vi "Image_Detect_Object.vi"(0 "Data":T3={"system"={"info"={"menuSelect"=0, "version"=0, "serial"="Test Sample", "captureActive"=FALSE, "captureBegin"=FALSE, "emptyAndRefill"=FALSE}, "userInfo"={"operatorName"="MRJ", "date"=timestamp(2713993200 s since 1904-01-01)}, "camera"={"exposureTime"=1, "aperture"=enum."Item 0", "framerate"=1, "framerateMax"=500, "legacyAttributes"=FALSE}}, "connections"={"arduino"={"connection"="MRJ", "status"=FALSE, "openState"=FALSE, "emptyStart"=500}, "pump"={"connection"="MRJ", "status"=FALSE, "command"="", "dispenseSpeed"=500, "flushSize"=100}, "camera"={"cam1"={"connection"="", "status"=FALSE}, "cam2"={"connection"="", "status"=FALSE}}}, "queue"={"process"={"cam1"=refnum, "cam2"=refnum, "queueSize"=0}, "save"={"cam1"=refnum, "cam2"=refnum, "queueSize"=0}, "overloadThreshold"=0}, "imageProcess"={"cam1"={"preAllocation"={"image"="Station", "originalDisplay"="Station", "originalRgb"="Station", "binary"="Station", "save"="Station", "calibrationFull"=refnum, "calibrationDetect"=refnum}, "calibration"={"pathFull"=path "C:/Users/au540322/Desktop/IHS_Project/images/Debris/Debris_0/Debris_0_2019_06_01-23-32-49-686.PNG", "pathDetect"=path "C:/Users/au540322/Desktop/IHS_Project/images/Debris/Debris_0/Debris_0_2019_06_01-23-32-49-686.PNG", "ROI"={"Left"=0, "Top"=0, "Right"=0, "Bottom"=0, "Rotation"=0.0}}}, "cam2"={"preAllocation"={"image"=refnum, "originalDisplay"=refnum, "originalRgb"=refnum, "binary"=refnum, "save"=refnum, "calibrationFull"=refnum, "calibrationDetect"=refnum}, "calibration"={"pathFull"=path "C:/Users/au540322/Desktop/IHS_Project/images/Debris/Debris_0/Debris_0_2019_06_01-23-32-49-686.PNG", "pathDetect"=path "C:/Users/au540322/Desktop/IHS_Project/images/Debris/Debris_0/Debris_0_2019_06_01-23-32-49-686.PNG", "ROI"={"Left"=0, "Top"=100, "Right"=100, "Bottom"=0, "Rotation"=0.0}}}, "process"={"planeExtract"=refnum, "planeSubtract"=refnum, "cropMask"=refnum}, "detection"={"sampleTimeout"=200, "sizeThreshold"=500, "detectionRegionPct"=0.0}}, "sampleData"={"sampleId"="", "projectId"="", "voucherID"="", "speciesName"="", "collectionDate"=timestamp(2713993200 s since 1904-01-01), "sampleStation"="", "location"="", "lat"=0.0, "lon"=0.0, "determiner"="", "sex"="", "otherNotes"=""}, "Session In"=""} {"sampleData"."collectionDate" format="%<%Y-%m-%d>T"; "imageProcess"."detection"."sizeThreshold" min=1; "imageProcess"."cam2"."calibration"."ROI"."Rotation" format="%.2f"; "imageProcess"."cam2"."calibration"."ROI"."Left" scale=0.0..1024.0; "imageProcess"."cam2"."calibration"."ROI"."Right" scale=0.0..1024.0; "imageProcess"."cam1"."calibration"."ROI"."Rotation" format="%.2f"; "imageProcess"."cam1"."calibration"."ROI"."Left" scale=0.0..1024.0; "imageProcess"."cam1"."calibration"."ROI"."Right" scale=0.0..1024.0; "queue"."overloadThreshold" min=1; "queue"."save"."queueSize" min=1; "queue"."process"."queueSize" min=1; "connections"."pump"."flushSize" min=1; "connections"."pump"."dispenseSpeed" min=1; "system"."camera"."framerateMax" min=1; "system"."userInfo"."date" format="%<%Y-%m-%dT%H:%M:%S+%z>T"; "system"."info"."version" items=["Standard", "XL"]; "system"."info"."menuSelect" items=["Session Data", "Extended Setup", "Buffer", "Camera", "Dispenser", "Stats", "Connections"]}, 5 "Image Pixels (U32)":u32[][](array[numeric]), 9 "Detect Crop":bool, 12 "Camera":T6=enum."Camera 2") -> (2 "error out":errorcluster, 3 "Obj Size":bool, 4 "Crop Image Out":T1(plugin-control), 6 "New image":T1(plugin-control), 8 "Image Binary":T1(plugin-control), 10 "Object Accept":bool, 14 "ROI descriptor":T2, 15 "Sample Data":dbl[](array[numeric]))   [LabVIEW 2022 SP3]
uses:
  <vilib>/vision/NI_Vision_Development_Module.lvlib
  Camera_ID.ctl
  <vilib>/userdefined/High Color/IMAQdx.ctl
  <vilib>/vision/Image Controls.llb/IMAQ Image.ctl
  controls/Data.ctl
panel:
  out "New image Blue plane":T1(plugin-control)
  out "Subtract":T1(plugin-control)
  in  "error in":errorcluster
  in  "Threshold":cluster{"Lower value":sgl, "Upper value":sgl}={"Lower value"=15.0, "Upper value"=256.0} {"Upper value" format="%.2f"; "Lower value" format="%.2f"}
  out "Calibration image in":T1(plugin-control)
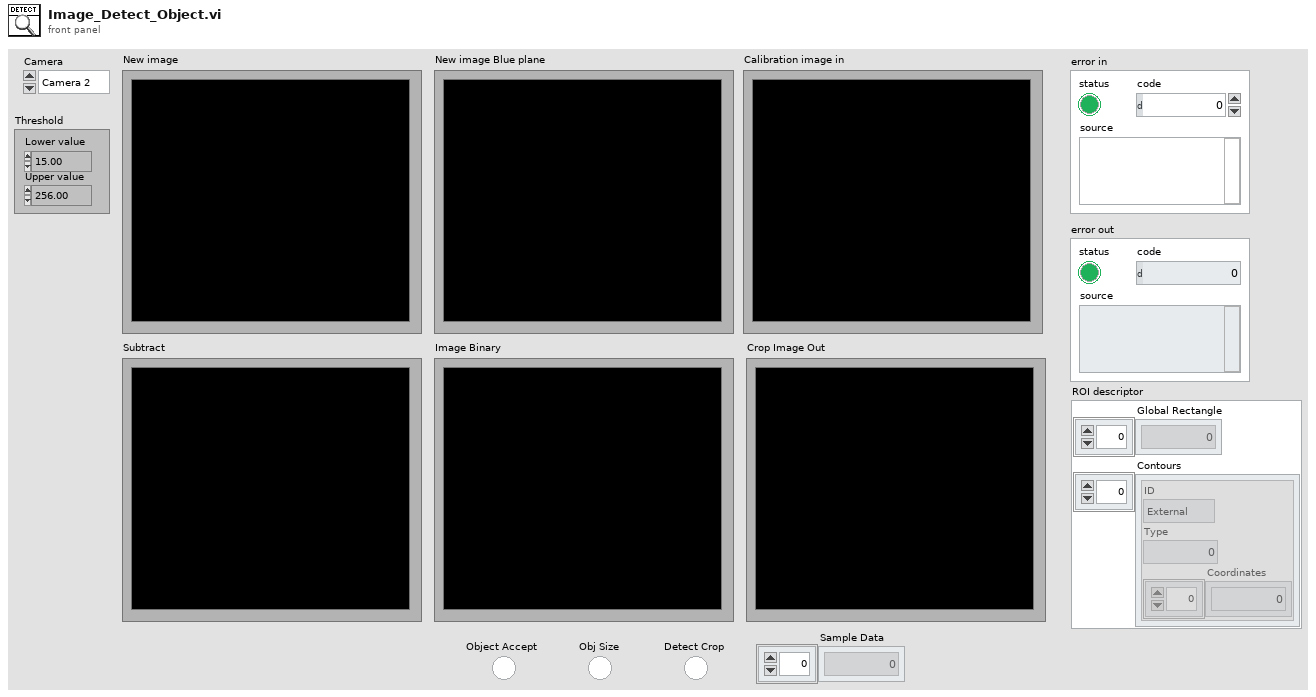
[diagram p1: front panel]
types:
  T1 = typedef "IMAQ Image.ctl" = refnum<image>
  T2 = cluster{"Global Rectangle":i32[], "Contours":cluster{"ID":enum32{"External", "Internal"}, "Type":u32, "Coordinates":i32[]}[]}
  T3 = typedef "Data.ctl" = cluster{"system":cluster{"info":cluster{"menuSelect":u16, "version":u16, "serial":string, "captureActive":bool, "captureBegin":bool, "emptyAndRefill":bool}, "userInfo":cluster{"operatorName":string, "date":timestamp}, "camera":cluster{"exposureTime":i32, "aperture":enum32{"Item 0", "Item 1", "Item 2", "Item 3"}, "framerate":i32, "framerateMax":i32, "legacyAttributes":bool}}, "connections":cluster{"arduino":cluster{"connection":refnum<visa-resource-name>, "status":bool, "openState":bool, "emptyStart":u32}, "pump":cluster{"connection":refnum<visa-resource-name>, "status":bool, "command":string, "dispenseSpeed":i32, "flushSize":i32}, "camera":cluster{"cam1":cluster{"connection":T4, "status":bool}, "cam2":cluster{"connection":T4, "status":bool}}}, "queue":cluster{"process":cluster{"cam1":refnum<queue>, "cam2":refnum<queue>, "queueSize":i32}, "save":cluster{"cam1":refnum<queue>, "cam2":refnum<queue>, "queueSize":i32}, "overloadThreshold":i32}, "imageProcess":cluster{"cam1":cluster{"preAllocation":cluster{"image":T1, "originalDisplay":T1, "originalRgb":T1, "binary":T1, "save":T1, "calibrationFull":T1, "calibrationDetect":T1}, "calibration":cluster{"pathFull":path, "pathDetect":path, "ROI":T5}}, "cam2":cluster{"preAllocation":cluster{"image":T1, "originalDisplay":T1, "originalRgb":T1, "binary":T1, "save":T1, "calibrationFull":T1, "calibrationDetect":T1}, "calibration":cluster{"pathFull":path, "pathDetect":path, "ROI":T5}}, "process":cluster{"planeExtract":T1, "planeSubtract":T1, "cropMask":T1}, "detection":cluster{"sampleTimeout":i32, "sizeThreshold":i32, "detectionRegionPct":dbl}}, "sampleData":cluster{"sampleId":string, "projectId":string, "voucherID":string, "speciesName":string, "collectionDate":timestamp, "sampleStation":string, "location":string, "lat":dbl, "lon":dbl, "determiner":string, "sex":string, "otherNotes":string}, "Session In":T4}
  T4 = typedef "IMAQdx.ctl" = refnum<k21>
  T5 = typedef "IMAQ Rectangle" = cluster{"Left":i32, "Top":i32, "Right":i32, "Bottom":i32, "Rotation":dbl}
  T6 = typedef "Camera_ID.ctl" = enum16{"Camera 1", "Camera 2"}
  T7 = typedef "Particle Parameters" = i32
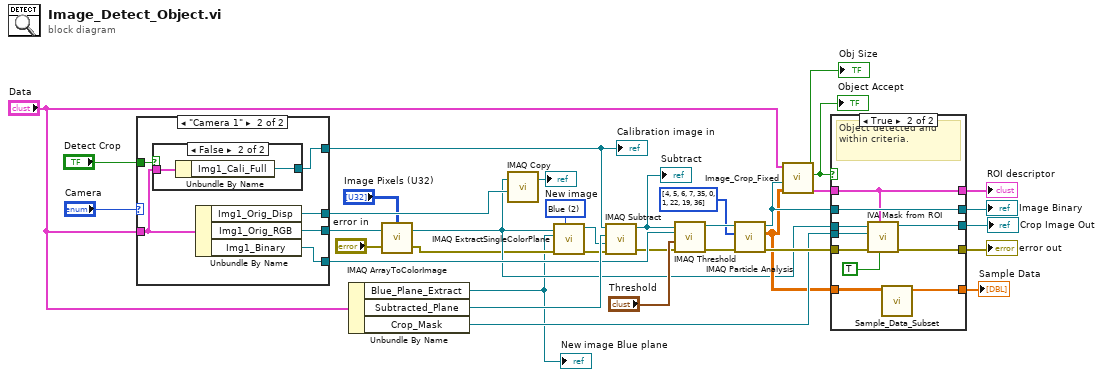
[diagram p0: block diagram]
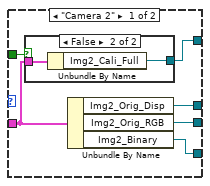
[diagram p2: hidden frame]
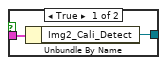
[diagram p3: hidden frame]
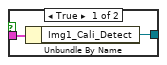
[diagram p4: hidden frame]
diagram:
  w17 = T7[] [4, 5, 6, 7, 35, 0, 1, 22, 19, 36] items=["Center of Mass X", "Center of Mass Y", "First Pixel X", "First Pixel Y", "Bounding Rect Left", "Bounding Rect Top", "Bounding Rect Right", "Bounding Rect Bottom", "Max Feret Diameter Start X", "Max Feret Diameter Start Y", "Max Feret Diameter End X", "Max Feret Diameter End Y", "Max Horiz. Segment Length Left", "Max Horiz. Segment Length Right", "Max Horiz. Segment Length Row", "-", "Bounding Rect Width", "Bounding Rect Height", "Bounding Rect Diagonal", "Perimeter", "Convex Hull Perimeter", "Holes' Perimeter", "Max Feret Diameter", "Equivalent Ellipse Major Axis", "Equivalent Ellipse Minor Axis", "Equivalent Ellipse Minor Axis (Feret)", "Equivalent Rect Long Side", "Equivalent Rect Short Side", "Equivalent Rect Diagonal", "Equivalent Rect Short Side (Feret)", "Average Horiz. Segment Length", "Average Vert. Segment Length", "Hydraulic Radius", "Waddel Disk Diameter", "-", "Area", "Holes' Area", "Particle & Holes' Area", "Convex Hull Area", "Image Area", "-", "Number of Holes", "Number of Horiz. Segments", "Number of Vert. Segments", "-", "Orientation", "Max Feret Diameter Orientation", "-", "% Area/Image Area", "% Area/(Particle & Holes' Area)", "Ratio of Equivalent Ellipse Axes", "Ratio of Equivalent Rect Sides", "-", "Elongation Factor", "Compactness Factor", "Heywood Circularity Factor", "Type Factor", "-", "Sum X", "Sum Y", "Sum XX", "Sum XY", "Sum YY", "Sum XXX", "Sum XXY", "Sum XYY", "Sum YYY", "-", "Moment of Inertia XX", "Moment of Inertia XY", "Moment of Inertia YY", "Moment of Inertia XXX", "Moment of Inertia XXY", "Moment of Inertia XYY", "Moment of Inertia YYY", "Norm. Moment of Inertia XX", "Norm. Moment of Inertia XY", "Norm. Moment of Inertia YY", "Norm. Moment of Inertia XXX", "Norm. Moment of Inertia XXY", "Norm. Moment of Inertia XYY", "Norm. Moment of Inertia YYY", "Hu Moment 1", "Hu Moment 2", "Hu Moment 3", "Hu Moment 4", "Hu Moment 5", "Hu Moment 6", "Hu Moment 7"] ("Pixel Measurements")
  w31 = 2 items=["Red", "Green", "Blue", "Hue", "Saturation", "Luminance", "Value", "Intensity"] ("Color Plane")
  n1 = case shown="\"Camera 1\"" "Camera" {
    tunnel: "Data" -> [w40 w50]
    tunnel: [w39 w49] -> w6
    tunnel: [w37 w48] -> w15
    tunnel: [w38 w46] -> w23
    tunnel: "Detect Crop" -> [w41 w51]
    tunnel: [w36 w47] -> w14
    frame "Camera 2" {
      n2 = case shown="False" w41 {
        tunnel: w40 -> [w43 w45]
        tunnel: [w42 w44] -> w39
        frame True {
          n3 = Unbundle By Name(w43) -> ("Img2_Cali_Detect"=w42:T1)
        }
        frame False {
          n4 = Unbundle By Name(w45) -> ("Img2_Cali_Full"=w44:T1)
        }
      }
      n5 = Unbundle By Name(w40) -> ("Img2_Orig_Disp"=w36:T1, "Img2_Orig_RGB"=w37:T1, "Img2_Binary"=w38:T1)
    }
    frame "Camera 1" {
      n6 = case shown="False" w51 {
        tunnel: w50 -> [w53 w55]
        tunnel: [w52 w54] -> w49
        frame True {
          n7 = Unbundle By Name(w53) -> ("Img1_Cali_Detect"=w52:T1)
        }
        frame False {
          n8 = Unbundle By Name(w55) -> ("Img1_Cali_Full"=w54:T1)
        }
      }
      n9 = Unbundle By Name(w50) -> ("Img1_Orig_Disp"=w47:T1, "Img1_Orig_RGB"=w48:T1, "Img1_Binary"=w46:T1)
    }
  }
  "Calibration image in" <- w6
  n10 = Unbundle By Name("Data") -> ("Blue_Plane_Extract"=w1:T1, "Subtracted_Plane"=w25:T1, "Crop_Mask"=w24:T1)
  "New image Blue plane" <- w1
  n11 = call "IMAQ ArrayToColorImage"("Image Pixels (U32)"="Image Pixels (U32)", "Image"=w15, "error in (no error)"="error in") -> ("Image Out"=w13:T1, "error out"=w8:errorcluster)  [unwired: 2 in]
  n12 = call "IMAQ Copy"("Image Dst"=w14, "Image Src"=w13) -> ("Image Dst Out"=→"New image":T1)  [unwired: 4 in, 1 out]
  n13 = call "IMAQ ExtractSingleColorPlane"("Color Plane"=w31, "error in (no error)"=w8, "Image Dst"=w1, "Image Src"=w13) -> ("error out"=w9:errorcluster, "Image Dst Out"=w5:T1)  [unwired: 6 out]
  n14 = call "IMAQ Subtract"("Image Src A"=w6, "Image Dst"=w25, "Image Src B"=w5, "error in (no error)"=w9) -> ("Image Dst Out"=w3:T1, "error out"=w10:errorcluster)  [unwired: 1 in, 2 out]
  "Subtract" <- w3
  n15 = call "IMAQ Threshold"("error in (no error)"=w10, "Range"="Threshold", "Image Dst"=w23, "Image Src"=w3) -> ("error out"=w28:errorcluster, "Image Dst Out"=w30:T1)  [unwired: 2 in, 4 out]
  n16 = call "IMAQ Particle Analysis"("error in (no error)"=w28, "Pixel Measurements"=w17, "Image"=w30) -> ("error out"=w32:errorcluster, "Particle Measurements (Pixels)"=w19:dbl[][], "Image Out (duplicate)"=w34:T1)  [unwired: 2 in, 4 out]
  n17 = call "Image_Crop_Fixed.vi"("Particle Measurements"=w19, "Image  in"=w34, "Data"="Data") -> ("ROI descriptor"=w35:T2, "Object accept"=w22:bool, "Object"=→"Obj Size":bool)  [unwired: 6 in]
  "Object Accept" <- w22
  n18 = case shown="True" w22 {
    tunnel: [w56 w67] -> w33
    tunnel: w32 -> [w57 w65]
    tunnel: [w58 w66] -> w2
    tunnel: w34 -> [w58 w66]
    tunnel: [w57 w64] -> w7
    tunnel: w35 -> [_ w59]
    tunnel: w24 -> [_ w60]
    tunnel: w13 -> [w56 w63]
    tunnel: w19 -> [_ w62]
    tunnel: [_ w61] -> w18
    tunnel: [_ w59] -> w11
    frame False {
      # "No object found or not within criteria."
    }
    frame True {
      # "Object detected and within criteria."
      n19 = call <vilib>:"IVA Mask from ROI.vi"("Shrink"=TRUE, "ROI Descriptor"=w59, "error in (no error)"=w65, 10:w60, "Image Src"=w63) -> ("error out"=w64:errorcluster, "Image Out"=w67:T1)  [unwired: 1 in, 4 out]
      n20 = call "Sample_Data_Subset.vi"("Particle Measurements (Pixels)"=w62) -> ("Sample Data"=w61:dbl[])  [unwired: 10 in]
    }
  }
  "Crop Image Out" <- w33
  "Image Binary" <- w2
  "error out" <- w7
  "Sample Data" <- w18
  "ROI descriptor" <- w11
